vi "GetSaveBandLevel.vi"(9 "Value in":u16, 11 "Task":enum16{"Read", "Save"}(ring)) -> (1 "Value out":u16)   [LabVIEW 2022 SP3]
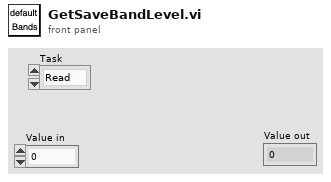
[diagram p1: front panel]
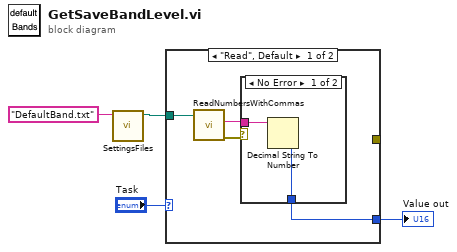
[diagram p0: block diagram]
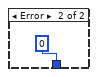
[diagram p2: hidden frame]
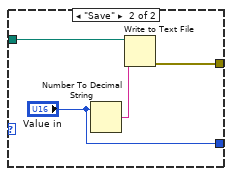
[diagram p3: hidden frame]
diagram:
  n1 = call "SettingsFiles.vi"("settings file name"="DefaultBand.txt" ("name or relative path")) -> ("file path"=w1:path)  [unwired: 9 in, 1 out]
  n2 = case shown="\"Read\", Default" "Task" {
    tunnel: w1 -> [w5 w15]
    tunnel: [_ w13] -> _
    tunnel: [w8 "Value in"] -> w3
    frame "Read", Default {
      n3 = call "ReadNumbersWithCommas.vi"("file (use dialog)"=w5) -> ("error out"=w7:errorcluster, "text"=w6:string)  [unwired: 7 in, 2 out]
      n4 = case shown="No Error" w7 {
        tunnel: w6 -> [w10 _]
        tunnel: [w9 0] -> w8
        frame No Error {
          n5 = Decimal String To Number(string=w10) -> (number=w9:i32)  [unwired: 2 in, 1 out]
        }
        frame Error {
        }
      }
    }
    frame "Save" {
      n6 = Number To Decimal String(number="Value in") -> (decimal integer string=w14:string)  [unwired: 1 in]
      n7 = Write to Text File(file (use dialog)=w15, text=w14) -> (error out=w13:errorcluster)  [unwired: 2 in, 2 out]
    }
  }
  "Value out" <- w3
